vi "LHF.DB.Mongo.Daemon.Shutdown.vi"(7 "timeout":i32=500, 8 "error in (no error)":errorcluster, 11 "LHF.DB.Mongo in":refnum<class "LHF.DB.Mongo.lvclass">) -> (0 "error out":errorcluster, 3 "LHF.DB.Mongo out":refnum<class "LHF.DB.Mongo.lvclass">)   [LabVIEW 2013, in "LHF.DB.Mongo.lvclass"]
doc: "Shutdown Daemon."
uses:
  LHF.DB.Mongo.lvclass
  LHF.DB.Mongo.lvclass/LHF.DB.Mongo.ctl
  C:/Users/Ricardo/Desktop/Projetos/LabVIEW-MongoDB/src/Driver/MongoDB.Driver.dll
  LabVIEW-MongoDB/src/Driver/MongoDB.Driver.dll
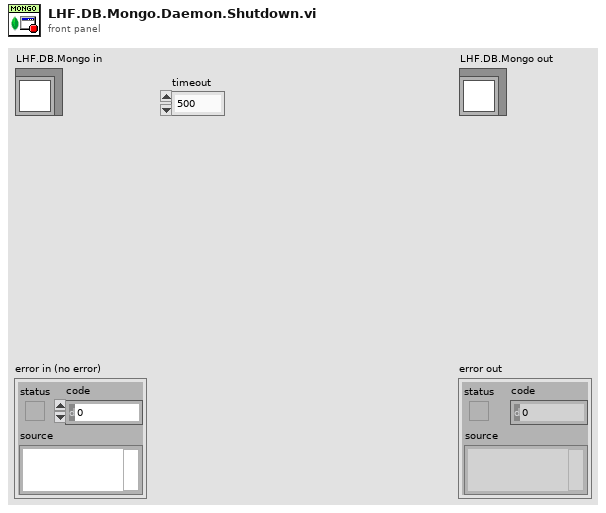
[diagram p1: front panel]
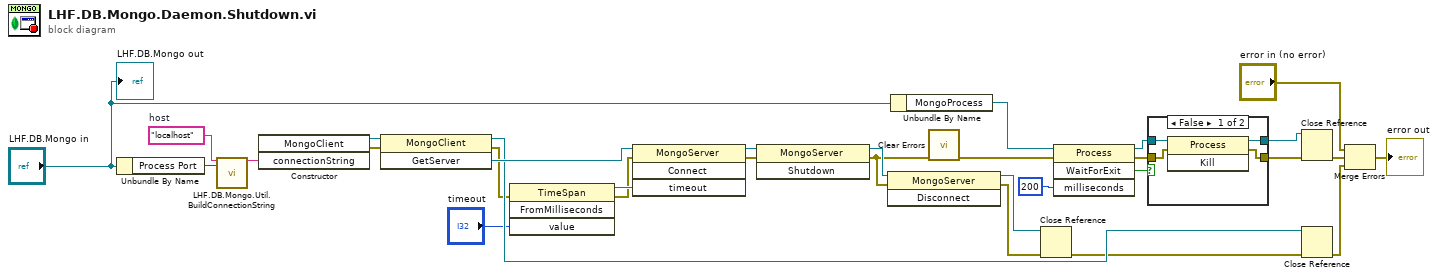
[diagram p0: block diagram]
diagram:
  w2 = "localhost"  # host
  n1 = Unbundle By Name("LHF.DB.Mongo in") -> ("Process Port"=w16:u32)
  n2 = call "LHF.DB.Mongo.Util.BuildConnectionString.vi"("host"=w2, "port"=w16) -> ("connectionString"=w10:string)  [unwired: 17 in]
  n3 = constructor class="MongoClient"("connectionString"=w10) -> (reference out=w24:refnum<k24>, error out=w25:errorcluster)  [unwired: 3 in, 2 out]
  n4 = invoke class="MongoClient" method="GetServer"(reference=w24, error in=w25) -> (reference out=w19:refnum<k24>, error out=w7:errorcluster, "GetServer"=w23:refnum<k24>)  [unwired: 1 in]
  n5 = invoke class="TimeSpan" method="FromMilliseconds"(error in=w7, "value"="timeout") -> (reference out=w9:refnum<k24>, error out=w6:errorcluster)  [unwired: 2 in, 2 out]
  n6 = invoke class="MongoServer" method="Connect"(reference=w23, error in=w6, "timeout"=w9) -> (reference out=w22:refnum<k24>, error out=w3:errorcluster)  [unwired: 1 in, 2 out]
  n7 = invoke class="MongoServer" method="Shutdown"(reference=w22, error in=w3) -> (reference out=w21:refnum<k24>, error out=w1:errorcluster)  [unwired: 1 in, 1 out]
  n8 = invoke class="MongoServer" method="Disconnect"(reference=w21, error in=w1) -> (reference out=w20:refnum<k24>, error out=w17:errorcluster)  [unwired: 1 in, 1 out]
  n9 = Unbundle By Name("LHF.DB.Mongo in") -> ("MongoProcess"=w29:refnum<k24>)
  n10 = call <vilib>:"Clear Errors.vi"("error in (no error)"=w1) -> ("error out"=w4:errorcluster)  [unwired: 6 in]
  n11 = Close Reference(reference=w20, error in (no error)=w17) -> (error out=w18:errorcluster)
  n12 = invoke class="Process" method="WaitForExit"(reference=w29, error in=w4, "milliseconds"=200) -> (reference out=w28:refnum<k24>, error out=w27:errorcluster, "WaitForExit"=w15:bool)  [unwired: 1 in, 1 out]
  n13 = case shown="False" w15 {
    tunnel: w28 -> [w35 w37]
    tunnel: w27 -> [w34 w36]
    tunnel: [w33 w37] -> w26
    tunnel: [w32 w36] -> w14
    frame False {
      n14 = invoke class="Process" method="Kill"(reference=w35, error in=w34) -> (reference out=w33:refnum<k24>, error out=w32:errorcluster)  [unwired: 1 in, 1 out]
    }
    frame True {
    }
  }
  n15 = Close Reference(reference=w26, error in (no error)=w14) -> (error out=w12:errorcluster)
  n16 = Close Reference(reference=w19, error in (no error)=w18) -> (error out=w13:errorcluster)
  n17 = Merge Errors("error in (no error)", w12, w13) -> (→"error out":errorcluster)
  "LHF.DB.Mongo out" <- "LHF.DB.Mongo in"
